vi "LimitAI16_src.vi"(0 "UnscaledAI":i16[](array[numeric])=[0, 0, 0, 0, 0, 0, 0, 0, 0, 0, 0, 0, 0, 0, 0, 0], 1 "LimitiEnabled":u16, 5 "HighLimit":i16[](array[numeric])=[0, 0, 0, 0, 0, 0, 0, 0, 0, 0, 0, 0, 0, 0, 0, 0], 7 "LowLimit":i16[](array[numeric])=[0, 0, 0, 0, 0, 0, 0, 0, 0, 0, 0, 0, 0, 0, 0, 0], 9 "UnscaledLimitHighIn":u16, 11 "UnscaledLimitLowIn":u16, 12 "ClearLimit":bool) -> (8 "LimitReached":bool, 10 "UnscaledLimitHighOut":u16, 15 "UnscaledLimitLowOut":u16)   [LabVIEW 2017]
doc: "Detects limits"
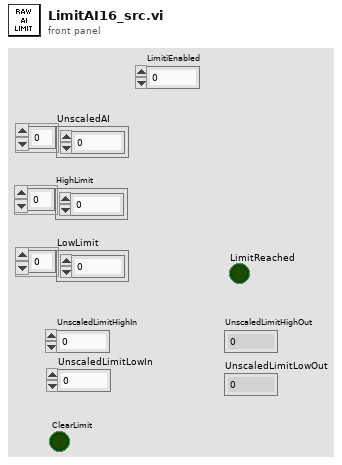
[diagram p1: front panel]
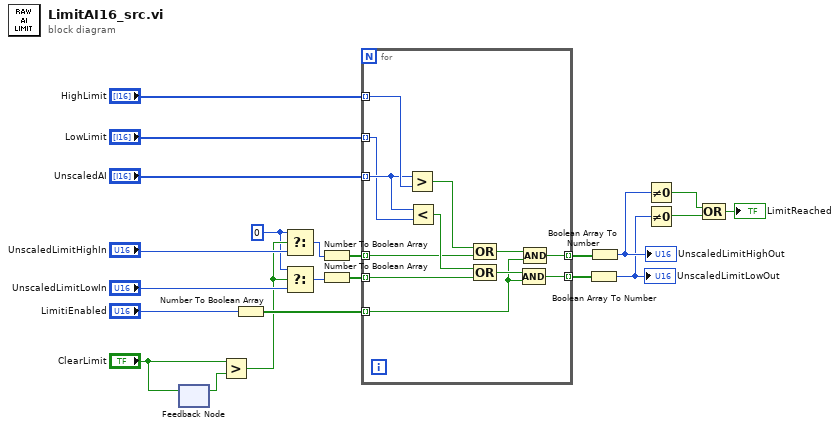
[diagram p0: block diagram]
diagram:
  w9 = u16 0 ("t")
  n1 = feedback-in #1("ClearLimit") -> ()
  n2 = feedback #1() -> (w11:bool)  [unwired: 1 in]
  n3 = Greater?(x="ClearLimit", y=w11) -> (0:w10:bool)
  n4 = Number To Boolean Array(number="LimitiEnabled") -> (Boolean array=w19:bool[])
  n5 = Select(t=w9, s=w10, f="UnscaledLimitHighIn") -> (s? t:f=w16:u16)
  n6 = Select(t=w9, s=w10, f="UnscaledLimitLowIn") -> (s? t:f=w15:u16)
  n7 = Number To Boolean Array(number=w16) -> (Boolean array=w21:bool[])
  n8 = Number To Boolean Array(number=w15) -> (Boolean array=w20:bool[])
  n9 = for {
    tunnel: "UnscaledAI" -> [w33] mode=indexing
    tunnel: "HighLimit" -> [w34] mode=indexing
    tunnel: "LowLimit" -> [w32] mode=indexing
    tunnel: w21 -> [w24] mode=indexing
    tunnel: w20 -> [w23] mode=indexing
    tunnel: w19 -> [w27] mode=indexing
    tunnel: [w26] -> w18 mode=indexing
    tunnel: [w25] -> w17 mode=indexing
    n10 = Greater?(x=w33, y=w34) -> (0:w31:bool)
    n11 = Less?(x=w33, y=w32) -> (x < y?=w30:bool)
    n12 = Compound Arithmetic op=OR(w31, w24) -> (w29:bool)
    n13 = Compound Arithmetic op=OR(w30, w23) -> (w28:bool)
    n14 = Compound Arithmetic op=AND(w28, w27) -> (w25:bool)
    n15 = Compound Arithmetic op=AND(w29, w27) -> (w26:bool)
  }
  n16 = Boolean Array To Number(Boolean array=w17) -> (number=w4:u16)
  "UnscaledLimitLowOut" <- w4
  n17 = Boolean Array To Number(Boolean array=w18) -> (number=w5:u16)
  "UnscaledLimitHighOut" <- w5
  n18 = Not Equal To 0?(x=w5) -> (x != 0?=w3:bool)
  n19 = Not Equal To 0?(x=w4) -> (x != 0?=w2:bool)
  n20 = Compound Arithmetic op=OR(w3, w2) -> (→"LimitReached":bool)
